vi "Model Sine Wave.vi"(6 "sampling info":cluster{"Fs":dbl, "#s":dbl}={"Fs"=1000.0, "#s"=1000.0} {"Fs" format="%.2p"}, 11 "Frequency":dbl) -> (2 "Sine wave":dbl[](array[numeric]), 3 "Waveform":waveform(dbl))   [LabVIEW 2020]
panel:
  out "Waveform Graph":waveform(dbl)(graph)
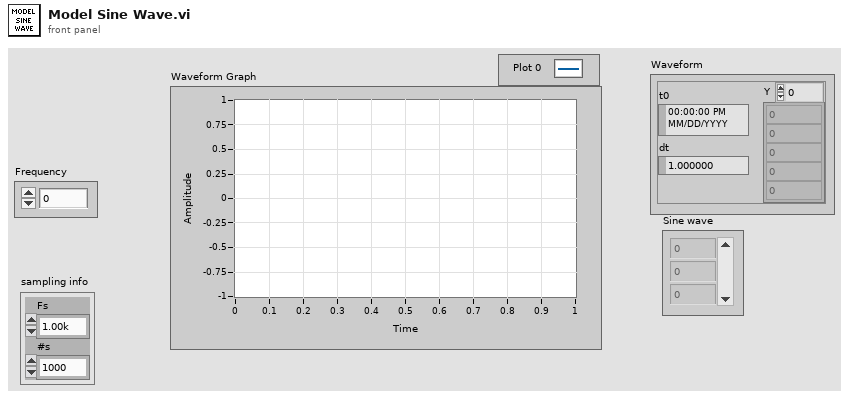
[diagram p1: front panel]
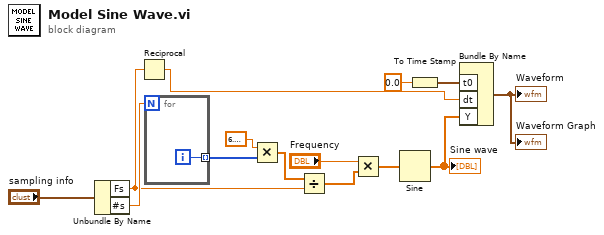
[diagram p0: block diagram]
diagram:
  n1 = Unbundle By Name("sampling info") -> ("Fs"=w6:dbl, "#s"=w13:dbl)
  n2 = Reciprocal(x=w6) -> (1/x=w3:dbl)
  n3 = for {
    N: w13 -> [_]
    tunnel: [w15] -> w12 mode=indexing
    i -> [w15]
  }
  n4 = Multiply(x=6.283185307179586, y=w12) -> (x*y=w9:dbl[])
  n5 = Divide(x=w9, y=w6) -> (x/y=w11:dbl[])
  n6 = Multiply(x="Frequency", y=w11) -> (x*y=w7:dbl[])
  n7 = Sine(x=w7) -> (sin(x)=w2:dbl[])
  "Sine wave" <- w2
  n8 = To Time Stamp(1:0.0) -> (0:w4:timestamp)
  n9 = Bundle By Name("t0"=w4, "dt"=w3, "Y"=w2) -> (→"Waveform Graph" →"Waveform":waveform(dbl))  [unwired: 1 in]
